vi "Set Configuration File List Names.vi"(8 "error in (no error)":errorcluster, 10 "Values":string[](array[string]), 11 "UI in":refnum<class "UI.lvclass">) -> (0 "error out":errorcluster)   [LabVIEW 2020, in "AR Example.lvlib" / "UI.lvclass"]
uses:
  UI.lvclass
  UI.lvclass/UI.ctl
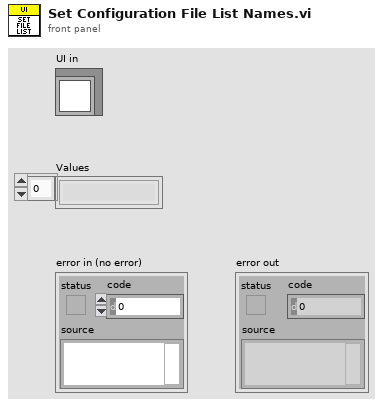
[diagram p1: front panel]
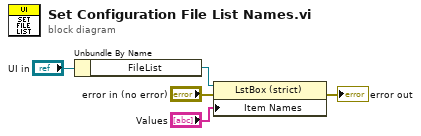
[diagram p0: block diagram]
diagram:
  n1 = Unbundle By Name("UI in") -> ("FileList"=w4:refnum<vi>)
  n2 = property class="LstBox (strict)"(reference=w4, error in="error in (no error)", "Item Names"="Values") -> (error out=→"error out":errorcluster)  [unwired: 1 out]
